vi "ScaleAndReplaceAcquiredData.vi"(6 "Type":T1, 7 "Lookup":variant, 8 "error in (no error)":errorcluster, 9 "Unscaled Data":u8[](array[numeric]), 10 "ID":u32, 11 "VS Data":dbl[](array[numeric])) -> (0 "error out":errorcluster, 3 "VS Data":dbl[](array[numeric]))   [LabVIEW 2015, in "Diagnostics Addon Engine.lvlib"]
uses:
  Diagnostics Addon Engine.lvlib
  Shared/Types/MessageType Selector.ctl
  Shared/Types/Datatable Lookup Positions.ctl
  <vilib>/xnet/xnet.llb/XNET Convert (Frame Raw to Signal).vi
  Convert ID to Raw Data.vi
  Shared/SubVIs/GUID Lookup.vi
  Shared/Diagnostics Addon Shared.lvlib
  <vilib>/NI Veristand/Custom Device Tools/Custom Device Utility Library/Custom Device Utility Library.lvlib
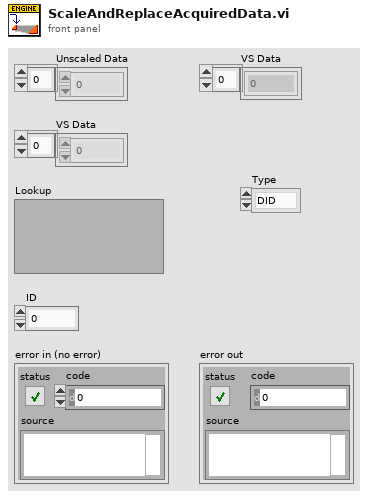
[diagram p1: front panel]
types:
  T1 = typedef "Diagnostics Addon Shared.lvlib/MessageType Selector.ctl" = enum16{"DID", "CDID", "PID", "CPID", "Read Memory", "Write Memory", "DTC Control", "IO Cmd", "IO Resp", "Routine Start Cmd", "Routine Start Resp", "Routine Request Cmd", "Routine Request Resp", "Routine Stop Cmd", "Routine Stop Resp"}
  T2 = typedef "Diagnostics Addon Shared.lvlib/Datatable Lookup Positions.ctl" = cluster{"Offset":i32, "Length":i32, "ByteLength":u16}
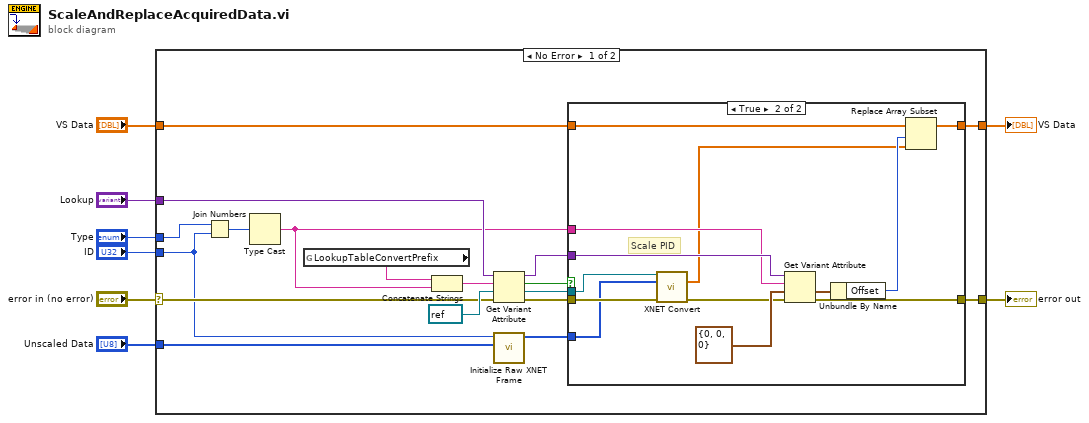
[diagram p0: block diagram]
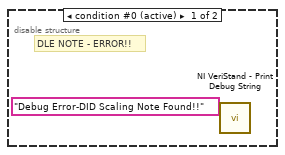
[diagram p3: hidden frame]
diagram:
  n1 = case shown="No Error" "error in (no error)" {
    selector: "error in (no error)" -> [w12 w44]
    tunnel: "VS Data" -> [w26 w43]
    tunnel: [w25 w43] -> w7
    tunnel: "Lookup" -> [w23 _]
    tunnel: [w14 w44] -> w5
    tunnel: "Unscaled Data" -> [w13 _]
    tunnel: "ID" -> [w11 _]
    tunnel: "Type" -> [w10 _]
    frame No Error {
      n2 = Join Numbers(hi=w10, lo=w11) -> ((hi.lo)=w9:u64)
      n3 = Type Cast(x=w9) -> (*(type *) &x=w16:string)  [unwired: 1 in]
      n4 = global read "GUID Lookup.vi" "LookupTableConvertPrefix"() -> (w24:string)
      n5 = Concatenate Strings(w24, w16) -> (w21:string)
      n6 = Get Variant Attribute(Variant=w23, name=w21, default value (empty Variant)=refnum<k21> refnum ("DID Conversion"), error in=w12) -> (duplicate Variant=w17:variant, found=w15:bool, value=w19:refnum<k21>, error out=w22:errorcluster)
      n7 = call "Initialize Raw XNET Frame.vi"("Data"=w13, "identifier"=w11) -> ("Raw Frame"=w18:u8[])  [unwired: 9 in]
      n8 = case shown="True" w15 {
        tunnel: w26 -> [w28 w40]
        tunnel: [w28 w39] -> w25
        tunnel: [w27 w37] -> w14
        tunnel: w22 -> [w27 w36]
        tunnel: w19 -> [_ w35]
        tunnel: w18 -> [_ w34]
        tunnel: w17 -> [_ w33]
        tunnel: w16 -> [_ w32]
        frame False {
          n9 = disable-structure shown="Default" {
            frame condition #0 (active) {
              # "DLE NOTE - ERROR!!"
              n10 = call <vilib>:"NI VeriStand - Print Debug String.vi"("Message"="Debug Error-DID Scaling Note Found!!" ("Debug String")) -> ()  [unwired: 10 in, 1 out]
            }
            frame condition #1 {
            }
          }
        }
        frame True {
          # "Scale PID"
          n11 = call-poly <vilib>:"XNET Convert.vi"("session in"=w35, "frame data"=w34, "error in (no error)"=w36) -> ("signal data"=w30:dbl[], "error out"=w38:errorcluster)  [unwired: 10 in, 1 out]
          n12 = Get Variant Attribute(Variant=w33, name=w32, default value (empty Variant)=T2 {"Offset"=0, "Length"=0, "ByteLength"=0} ("cluster"), error in=w38) -> (value=w42:T2, error out=w37:errorcluster)  [unwired: 2 out]
          n13 = Unbundle By Name(w42) -> ("Offset"=w31:i32)
          n14 = Replace Array Subset(array=w40, new element=w30, index=w31) -> (w39:dbl[])
        }
      }
    }
    frame Error {
    }
  }
  "VS Data" <- w7
  "error out" <- w5
